vi "Test Fail if Expected Call Not Made.vi"(8 "error in (no error)":errorcluster, 11 "Test Case In":refnum<class "One or More Expectation Test.lvclass">) -> (0 "error out":errorcluster, 3 "Test Case Out":refnum<class "One or More Expectation Test.lvclass">)   [LabVIEW 2020, in "One or More Expectation Test.lvclass"]
uses:
  One or More Expectation Test.lvclass
  C:/Program Files (x86)/National Instruments/LabVIEW 2020/vi.lib/Astemes/LUnit/Test Case.lvclass
  Test Interface Mock/Test Interface Mock.lvclass
  C:/git/astemes-lmock/sandbox/Mock/Mock.lvclass
  Expectation Test/Expectation Test.lvclass
  One or More of/One Of/One or More.lvclass
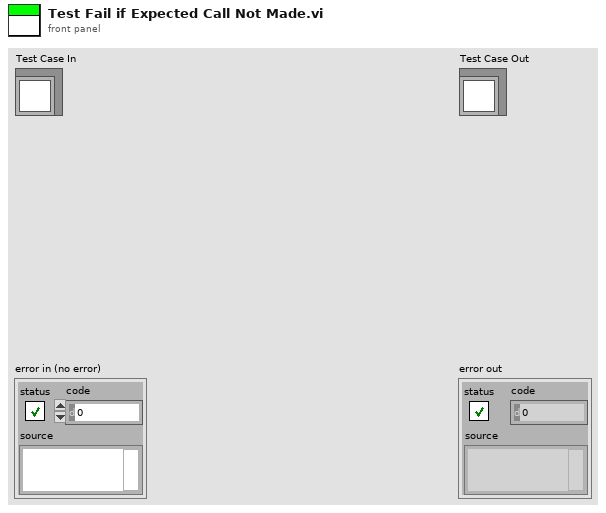
[diagram p1: front panel]
types:
  T1 = enum16{"", "Passed", "Failed", "Error", "Skipped", "Setup Error", "Broken", "Teardown Error"}
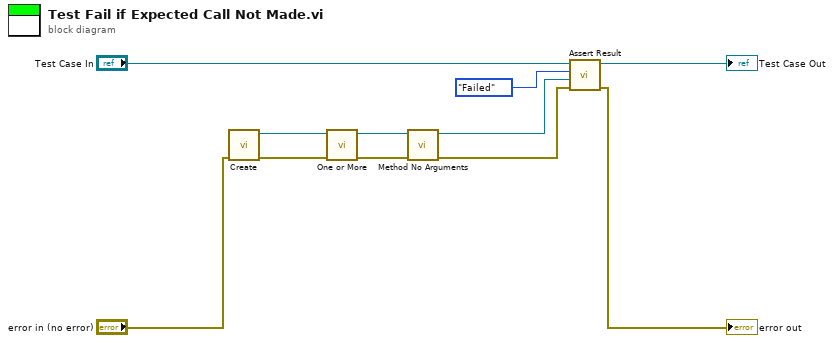
[diagram p0: block diagram]
diagram:
  n1 = call "Create.vi"("error in (no error)"="error in (no error)") -> ("error out"=w7:errorcluster, "Test Interface Mock Out"=w5:refnum<class "Test Interface Mock.lvclass">)  [unwired: 9 in]
  n2 = call "One or More.vi"("error in (no error)"=w7, "Mock in"=w5) -> ("error out"=w6:errorcluster, "Mock out"=w4:refnum<class "Test Interface Mock.lvclass">)  [unwired: 8 in]
  n3 = call-dynamic "Method No Arguments.vi"("error in (no error)"=w6, "Mock In"=w4) -> ("error out"=w2:errorcluster, "Mock Out"=w3:refnum<class "Test Interface Mock.lvclass">)  [unwired: 8 in]
  n4 = call "Assert Result.vi"("error in (no error)"=w2, "Mock"=w3, "Status"=T1."Failed", "LUnit Test Case In"="Test Case In") -> ("error out"=→"error out":errorcluster, "LUnit Test Case Out"=→"Test Case Out":refnum<class "One or More Expectation Test.lvclass">)  [unwired: 6 in]
